vi "HGF_SVVarManVisitor_delete.appendData2Variant.vi"(0 "variant":variant, 2 "Shared Variable":refnum<k21>, 3 "return-to Event":refnum<class "HGF_TriggeredEvent.lvclass">, 5 "error in":errorcluster) -> (14 "dup variant":variant, 19 "error out":errorcluster)   [LabVIEW 2012, in "HGF_SV.lvlib" / "HGF_SVVarManVisitor_delete.lvclass"]
uses:
  HGF_SVVarManVisitor_delete.lvclass
  HGF_BaseClasses/HGF_TriggeredEvent/HGF_TriggeredEvent.lvclass
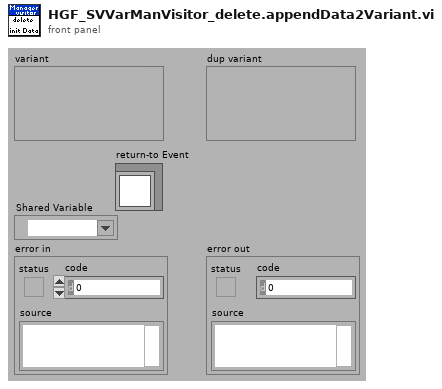
[diagram p1: front panel]
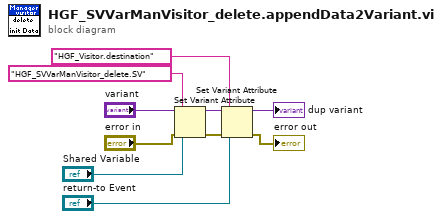
[diagram p0: block diagram]
diagram:
  n1 = Set Variant Attribute(Variant="variant", name="HGF_SVVarManVisitor_delete.SV", value="Shared Variable", error in="error in") -> (Variant out=w5:variant, error out=w7:errorcluster)  [unwired: 1 out]
  n2 = Set Variant Attribute(Variant=w5, name="HGF_Visitor.destination", value="return-to Event", error in=w7) -> (Variant out=→"dup variant":variant, error out=→"error out":errorcluster)  [unwired: 1 out]
